vi "Single Analog DAQmx Task (SubVI).vi"(0 "Module Configure":T1={"DAQ #"=1, "Module #"=4, "Samples"=1000, "Mode"=10178, "Rate (Hz)"=1000.0, "Min VDC"=-10.0, "Max VDC"=32.0, "Module Type"=enum."CDAQ"} {"Rate (Hz)" format="%0.2f"; "Mode" items=["Finite Samples"=10178, "Continuous Samples"=10123, "Hardware Timed Single Point"=12522]}, 1 "E-STOP Input":bool) -> (2 "Task OUT":refnum<k21>="cDAQ1Mod4", 3 "Waveform Output":waveform(dbl), 4 "Error OUT":errorcluster)   [LabVIEW 2009]
uses:
  <vilib>/DAQmx/configure/timing.llb/DAQmx Timing (Sample Clock).vi
  <vilib>/DAQmx/create/channels.llb/DAQmx Create Channel (AI-Voltage-Basic).vi
  <vilib>/DAQmx/read.llb/DAQmx Read (Analog Wfm 1Chan NSamp).vi
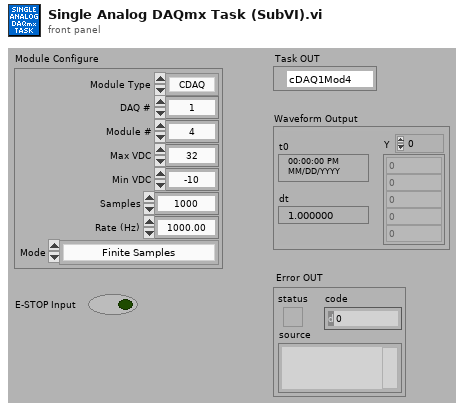
[diagram p1: front panel]
types:
  T1 = cluster{"DAQ #":i32, "Module #":i32, "Samples":i32, "Mode":i32, "Rate (Hz)":dbl, "Min VDC":dbl, "Max VDC":dbl, "Module Type":enum16{"CDAQ", "SCXI"}}
  T2 = cluster{"DAQ #":bool, "Module #":bool, "Samples":bool, "Mode":bool, "Rate (Hz)":bool, "Min VDC":bool, "Max VDC":bool, "Module Type":bool}
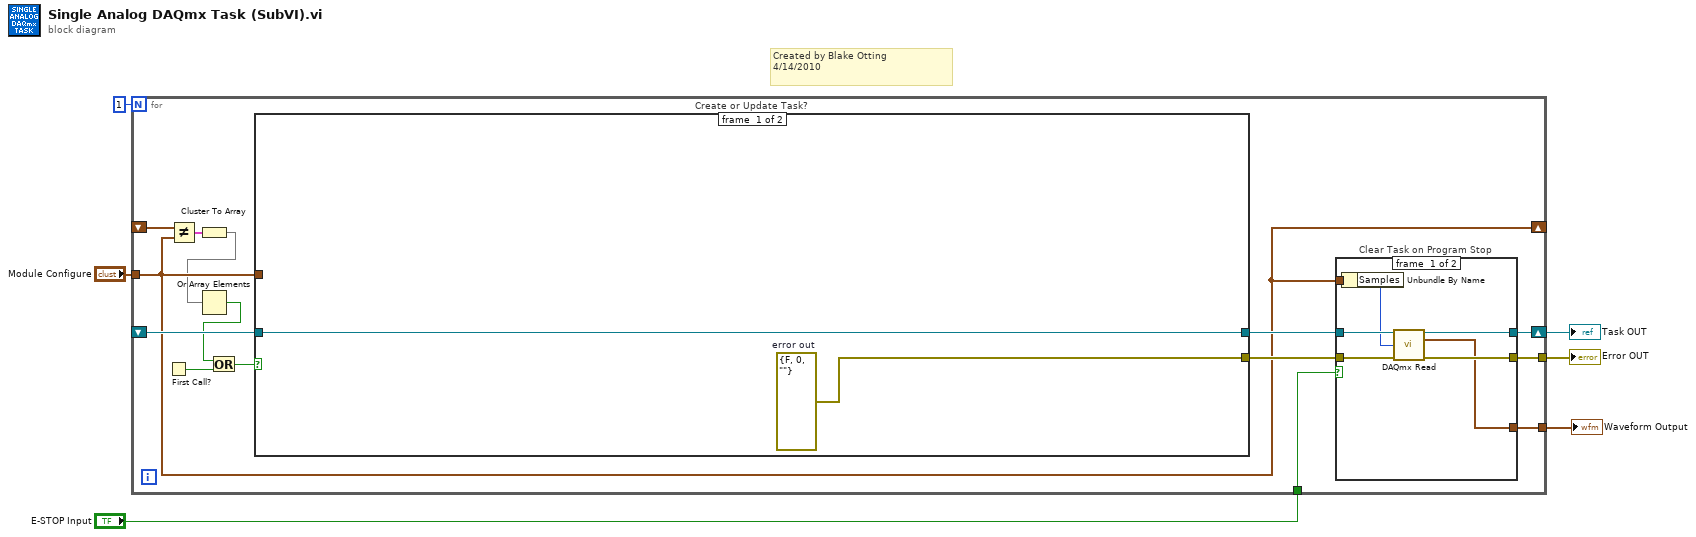
[diagram p0: block diagram]
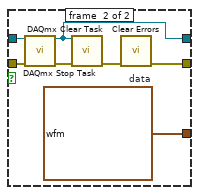
[diagram p2: hidden frame]
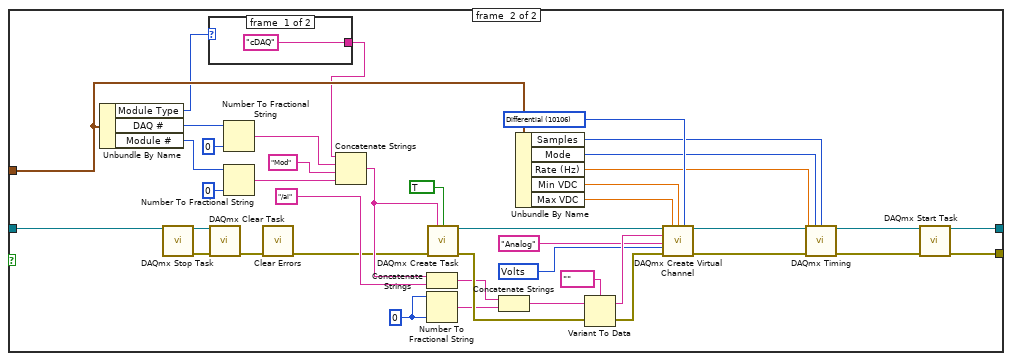
[diagram p3: hidden frame]
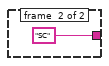
[diagram p4: hidden frame]
diagram:
  # "Created by Blake Otting\n4/14/2010"
  n1 = for {
    N: 1 -> [_]
    tunnel: "Module Configure" -> [w8]
    tunnel: [w15] -> w2
    shift-right: [w16] -> w3
    shift-left: _ -> [w20]
    tunnel: "E-STOP Input" -> [w17]
    tunnel: [w14] -> w6
    shift-right: [w8] -> _
    shift-left: _ -> [w13]
    n2 = First Call?() -> (First Call?: T/F=w11:bool)
    n3 = Not Equal?(x=w13, y=w8) -> (x != y?=w12:T2)
    n4 = Cluster To Array(cluster=w12) -> (array=w7:bool[])
    n5 = Or Array Elements(Boolean array=w7) -> (logical OR=w9:bool)
    n6 = Or(x=w9, y=w11) -> (x .or. y?=w10:bool)
    n7 = case "Create or Update Task?" shown="True" w10 {
      tunnel: [w35 w55] -> w19
      tunnel: [w36 w54] -> w18
      tunnel: w8 -> [_ w49]
      tunnel: w20 -> [w35 w40]
      frame #0 {
        w36 = errorcluster {"status"=FALSE, "code"=0, "source"=""}  # error out
      }
      frame #1 {
        w52 = 10106 items=["default"=-1, "RSE"=10083, "NRSE"=10078, "Differential"=10106, "Pseudodifferential"=12529] ("input terminal configuration")
        w53 = 10348 items=["Volts"=10348, "From Custom Scale"=10065] ("units")
        w50 = i16 0 ("precision (6)")
        n8 = Unbundle By Name(w49) -> ("Module Type"=w43:enum16{"CDAQ", "SCXI"}, "DAQ #"=w71:i32, "Module #"=w70:i32)
        n9 = call <vilib>:"DAQmx Stop Task.vi"("task/channels in"=w40) -> ("task out"=w41:refnum<k21>, "error out"=w39:errorcluster)  [unwired: 13 in]
        n10 = case shown="\"SCXI\"" w43 {
          tunnel: ["cDAQ" ("physical channel") "SC" ("physical channel")] -> w42
          frame #0 {
          }
          frame #1 {
          }
        }
        n11 = call <vilib>:"DAQmx Clear Task.vi"("task in"=w41, "error in"=w39) -> ("error out"=w38:errorcluster)  [unwired: 13 in]
        n12 = Number To Fractional String(number=w71, precision (6)=i16 0) -> (F-format string=w74:string)  [unwired: 2 in]
        n13 = Number To Fractional String(number=w70, precision (6)=i16 0) -> (F-format string=w72:string)  [unwired: 2 in]
        n14 = call <vilib>:"Clear Errors.vi"("error in (no error)"=w38) -> ("error out"=w37:errorcluster)  [unwired: 6 in]
        n15 = Concatenate Strings(w42, w74, "Mod" ("physical channel"), w72) -> (w66:string)
        n16 = Concatenate Strings(w66, "/ai" ("physical channel")) -> (w67:string)
        n17 = Number To Fractional String(number=w50, precision (6)=w50) -> (F-format string=w60:string)  [unwired: 2 in]
        n18 = call <vilib>:"DAQmx Create Task.vi"("new task name"=w66, "auto cleanup"=TRUE, "error in"=w37) -> ("task out"=w65:refnum<k21>, "error out"=w77:errorcluster)  [unwired: 11 in]
        n19 = Concatenate Strings(w67, w60) -> (w61:string)
        n20 = Unbundle By Name(w49) -> ("Samples"=w48:i32, "Mode"=w47:i32, "Rate (Hz)"=w46:dbl, "Min VDC"=w45:dbl, "Max VDC"=w44:dbl)
        n21 = Variant To Data(error in=w77, Variant=w61, type=tag "" ("physical channels")) -> (error out=w62:errorcluster, data=w64:tag)
        n22 = call-poly <vilib>:"DAQmx Create Virtual Channel.vi"("task in"=w65, "maximum value"=w44, "minimum value"=w45, "input terminal configuration"=w52, "physical channels"=w64, "name to assign"="Analog" ("string"), "units"=w53, "error in"=w62) -> ("task out"=w59:refnum<k21>, "error out"=w58:errorcluster)  [unwired: 6 in]
        n23 = call-poly <vilib>:"DAQmx Timing.vi"("task/channels in"=w59, "sample mode"=w47, "samples per channel"=w48, "rate"=w46, "error in"=w58) -> ("task out"=w57:refnum<k21>, "error out"=w56:errorcluster)  [unwired: 9 in]
        n24 = call <vilib>:"DAQmx Start Task.vi"("task/channels in"=w57, "error in"=w56) -> ("task out"=w55:refnum<k21>, "error out"=w54:errorcluster)  [unwired: 12 in]
      }
    }
    n25 = case "Clear Task on Program Stop" shown="True" w17 {
      tunnel: w18 -> [w25 w29]
      tunnel: [w24 w33] -> w15
      tunnel: w19 -> [w27 w32]
      tunnel: [w26 w31] -> w16
      tunnel: [w23 w28] -> w14
      tunnel: w8 -> [w22 _]
      frame #0 {
        n26 = Unbundle By Name(w22) -> ("Samples"=w21:i32)
        n27 = call-poly <vilib>:"DAQmx Read.vi"("task/channels in"=w27, "number of samples per channel"=w21, "error in"=w25) -> ("task out"=w26:refnum<k21>, "data"=w23:waveform(dbl), "error out"=w24:errorcluster)  [unwired: 10 in]
      }
      frame #1 {
        w28 = waveform(dbl) {"t0"=timestamp(0 s since 1904-01-01), "dt"=1.0, "Y"=[]}  # data
        n28 = call <vilib>:"DAQmx Stop Task.vi"("task/channels in"=w32, "error in"=w29) -> ("task out"=w31:refnum<k21>, "error out"=w30:errorcluster)  [unwired: 12 in]
        n29 = call <vilib>:"DAQmx Clear Task.vi"("task in"=w31, "error in"=w30) -> ("error out"=w34:errorcluster)  [unwired: 13 in]
        n30 = call <vilib>:"Clear Errors.vi"("error in (no error)"=w34) -> ("error out"=w33:errorcluster)  [unwired: 6 in]
      }
    }
  }
  "Error OUT" <- w2
  "Task OUT" <- w3
  "Waveform Output" <- w6
